vi "LiftControl2.vi"   [LabVIEW 2010]
uses:
  <vilib>/NXT/NXTIO Xnodes/AddressXNode/NXTIOAddress.xnode
  <vilib>/NXT/Subs/MotorXNode.DC Motor Type.ctl
  4150_RingItUp_State/4150 ringbot v1.lvrbt
  <vilib>/NXT/Subs/MotorXNode.2DCMotor.ctl
  <vilib>/NXT/Subs/LVHSConnector.ctl
  <vilib>/NXT/Block Support/NXT_ButtonSelector.ctl
  <vilib>/NXT/NXTIO Xnodes/NXTIOXNode/NXTIO.xnode
  <vilib>/NXT/Dual Mode Library/Sensors/readNXTButton.vi
  <vilib>/NXT/NXTIO Xnodes/NXTIONodeSubVIs/TETRIX IO Move DC Motors.vi
types:
  T1 = typedef "MotorXNode.DC Motor Type.ctl" = enum16{"DC Motor"}
  T2 = cluster{"DC Motor":T1, "Address":i16, "Address":i16}
  T3 = typedef "NXT_ButtonSelector.ctl" = u16
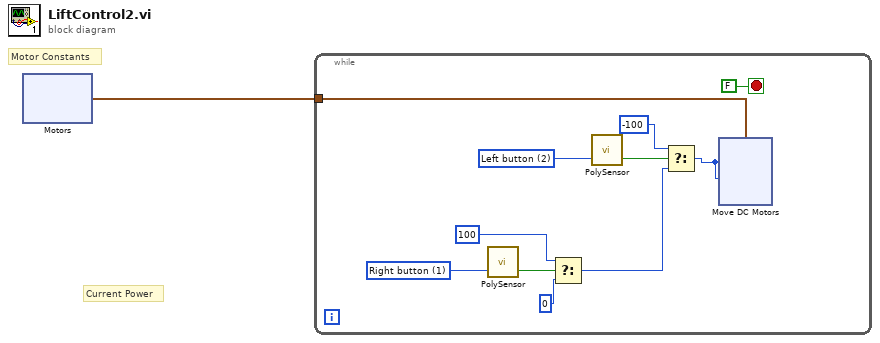
[diagram p0: block diagram]
diagram:
  # "Motor Constants"
  # "Current Power"
  n1 = xnode "Motors"() -> ("DC Motor"=w1:T2)
  n2 = while {
    tunnel: w1 -> [w6]
    stop <- FALSE stop-if-true
    w10 = T3 2 items=["Enter button"=3, "Left button"=2, "Right button"=1] ("Button (Enter button)")
    w11 = T3 1 items=["Enter button"=3, "Left button"=2, "Right button"=1] ("Button (Enter button)")
    n3 = call-poly <vilib>:"PolySensor.vi"("Button (Enter button)"=w11) -> ("Yes/No"=w8:bool)  [unwired: 2 in, 1 out]
    n4 = Select(t=i8 100 ("Power/Speed 1"), s=w8, f=i8 0) -> (s? t:f=w7:i8)
    n5 = call-poly <vilib>:"PolySensor.vi"("Button (Enter button)"=w10) -> ("Yes/No"=w9:bool)  [unwired: 2 in, 1 out]
    n6 = Select(t=i8 -100, s=w9, f=w7) -> (s? t:f=w2:i8)
    n7 = xnode "Move DC Motors"("Power/Speed 2"=w2, "Power/Speed 1"=w2, "Motors"=w6) -> ()  [unwired: 1 in, 1 out]
  }
